vi "SD-Read Registry Value Simple STR.vi"(6 "error in (no error)":errorcluster, 7 "default data":string, 8 "value":string, 9 "refnum":T1) -> (0 "error out":errorcluster, 1 "String/Binary data":string, 2 "simple data type":enum16{"String", "Binary", "DWORD"}(ring), 3 "refnum out":T1)   [LabVIEW 2020]
doc: "Reads data and the simplified data type from a registry value. If the key or value does not exist or an unrecoverable error occurs, the VI returns the default data. Wire data to the <B>default data</B> input to determine the polymorphic instance to use or manually select the instance."
uses:
  SD-Registry refnum.ctl
  SD-Read Registry Value STR.vi
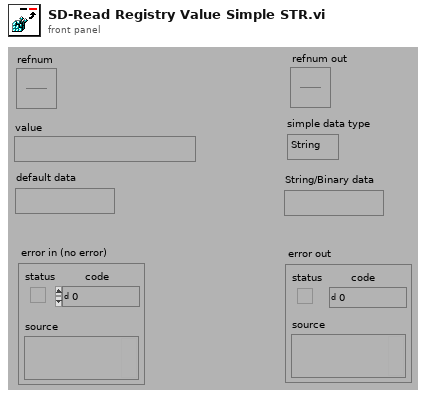
[diagram p1: front panel]
types:
  T1 = typedef "SD-Registry refnum.ctl" = refnum<k1>
  T2 = enum32{"REG_NONE", "REG_SZ", "REG_EXPAND_SZ", "REG_BINARY", "REG_DWORD_LITTLE_ENDIAN", "REG_DWORD_BIG_ENDIAN", "REG_LINK", "REG_MULTI_SZ", "REG_RESOURCE_LIST", "REG_FULL_RESOURCE_DESCRIPTOR", "REG_RESOURCE_REQUIREMENTS_LIST"}
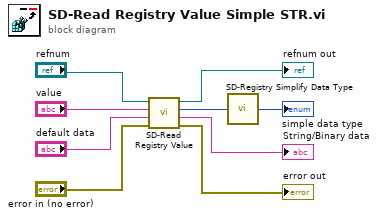
[diagram p0: block diagram]
diagram:
  n1 = call-poly "SD-Read Registry Value.vi"("error in (no error)"="error in (no error)", "default data"="default data", "value"="value", "refnum"="refnum") -> ("error out"=→"error out":errorcluster, "String/Binary data"=→"String/Binary data":string, "data type"=w2:T2, "refnum out"=→"refnum out":T1)  [unwired: 4 out]
  n2 = call "SD-Registry Simplify Data Type.vi"("data type"=w2) -> ("simple data type"=→"simple data type":enum16{"String", "Binary", "DWORD"})  [unwired: 4 out]
